vi "Machine State.vi"(11 "Numeric":i32) -> (3 "Profile Status":string)   [LabVIEW 2016, in "GEA2_Toolkit.lvlib"]
uses:
  library/GEA2_Toolkit.lvlib
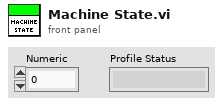
[diagram p1: front panel]
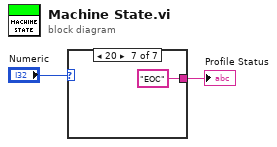
[diagram p0: block diagram]
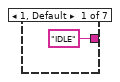
[diagram p2: hidden frame]
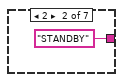
[diagram p3: hidden frame]
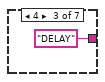
[diagram p4: hidden frame]
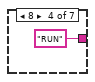
[diagram p5: hidden frame]
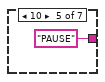
[diagram p6: hidden frame]
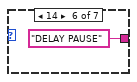
[diagram p7: hidden frame]
diagram:
  n1 = case shown="20" "Numeric" {
    tunnel: ["IDLE" "STANDBY" "DELAY" "RUN" "PAUSE" "DELAY PAUSE" ("Profile Status") "EOC"] -> w2
    frame 1, Default {
    }
    frame 2 {
    }
    frame 4 {
    }
    frame 8 {
    }
    frame 10 {
    }
    frame 14 {
    }
    frame 20 {
    }
  }
  "Profile Status" <- w2
